vi "Heat2D_Cal Tridiagonal.vi"(9 "Boundary Condition":cluster{"type":T4, "Value":dbl[][]}[](array[cluster]) {"type" items=["Dirichlet", "Neumann"]}, 10 "Coefficients":T2, 11 "Domain":T3={"t"={"initial t"=0.0, "final t"=1.0, "# of t-points"=11}, "x"={"start x"=0.0, "end x"=1.0, "# of x-points"=11}, "y"={"start y"=0.0, "end y"=1.0, "# of y-points"=11}}) -> (0 "X RHS":dbl[][](array[numeric]), 2 "Coefficients Dup":T2, 3 "TriDia Cluster":T1)   [LabVIEW 2017, in "NI_PDE.lvlib"]
uses:
  <vilib>/gmath/NI_PDE.lvlib
  <vilib>/gmath/pde.llb/Common/PDE_BC Type.ctl
  <vilib>/Analysis/NI_AALPro.lvlib
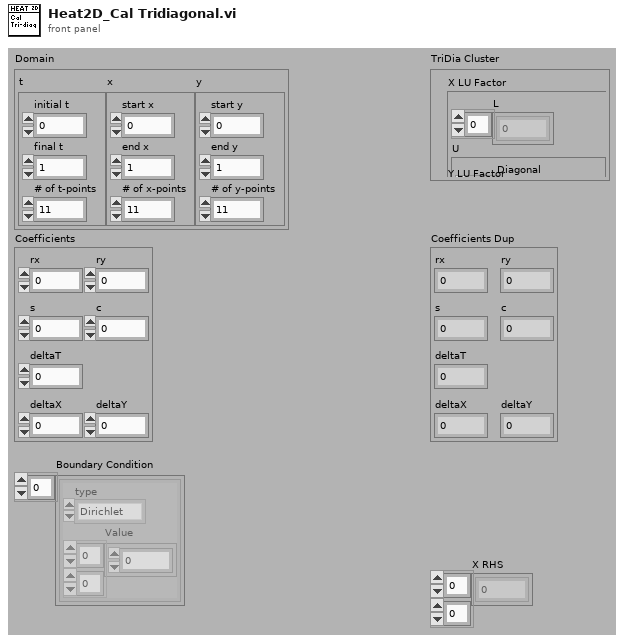
[diagram p1: front panel]
types:
  T1 = cluster{"X LU Factor":cluster{"L":dbl[], "U":cluster{"Diagonal":dbl[], "Super Diagonal":dbl[], "2nd Super Diagonal":dbl[]}, "Pivot":i32[]}, "Y LU Factor":cluster{"L":dbl[], "U":cluster{"Diagonal":dbl[], "Super Diagonal":dbl[], "2nd Super Diagonal":dbl[]}, "Pivot":i32[]}, "X Tridiagonal":cluster{"SubDiagonal":dbl[], "MainDiagonal":dbl[], "SuperDiagonal":dbl[]}, "Y Tridiagonal":cluster{"SubDiagonal":dbl[], "MainDiagonal":dbl[], "SuperDiagonal":dbl[]}}
  T2 = cluster{"rx":dbl, "ry":dbl, "s":dbl, "c":dbl, "deltaT":dbl, "deltaX":dbl, "deltaY":dbl}
  T3 = cluster{"t":cluster{"initial t":dbl, "final t":dbl, "# of t-points":i32}, "x":cluster{"start x":dbl, "end x":dbl, "# of x-points":i32}, "y":cluster{"start y":dbl, "end y":dbl, "# of y-points":i32}}
  T4 = typedef "NI_PDE.lvlib/PDE_BC Type.ctl" = i32
  T5 = cluster{"SubDiagonal":dbl[], "MainDiagonal":dbl[], "SuperDiagonal":dbl[]}
  T6 = cluster{"Diagonal":dbl[], "Super Diagonal":dbl[], "2nd Super Diagonal":dbl[]}
  T7 = cluster{"L":dbl[], "U":cluster{"Diagonal":dbl[], "Super Diagonal":dbl[], "2nd Super Diagonal":dbl[]}, "Pivot":i32[]}
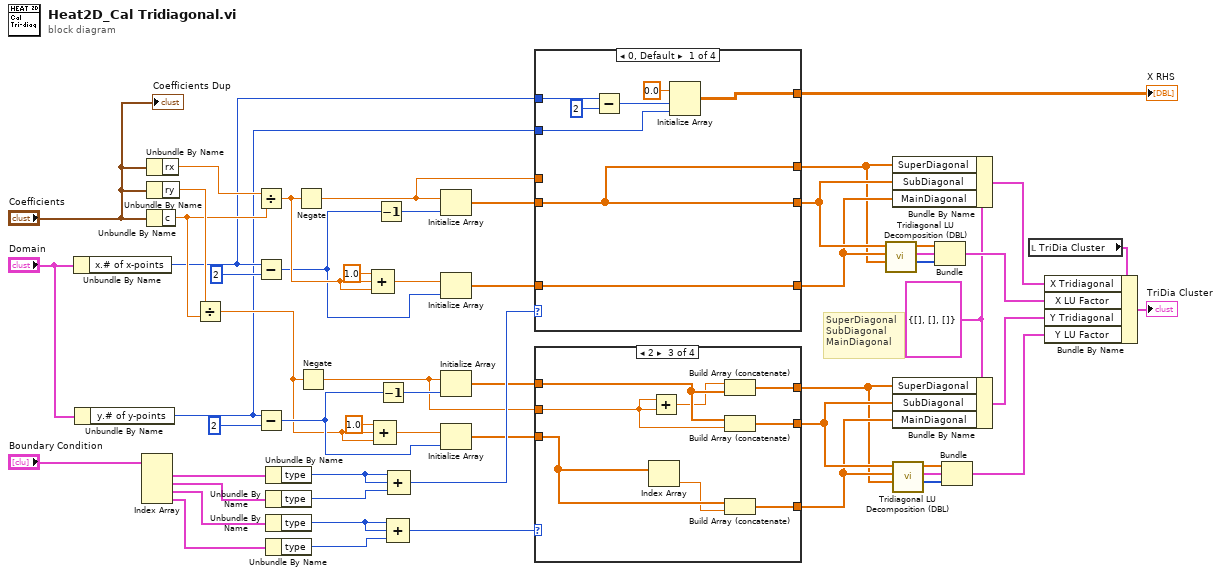
[diagram p0: block diagram]
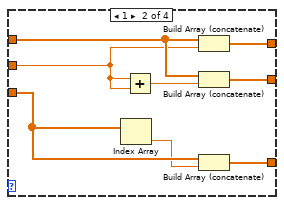
[diagram p3: hidden frame]
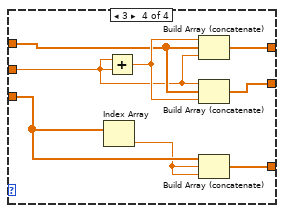
[diagram p4: hidden frame]
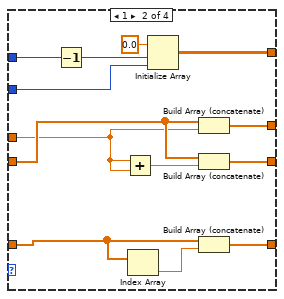
[diagram p5: hidden frame]
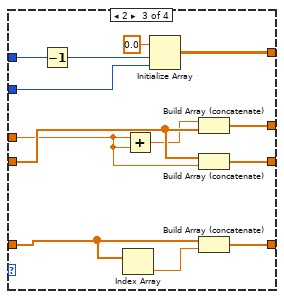
[diagram p6: hidden frame]
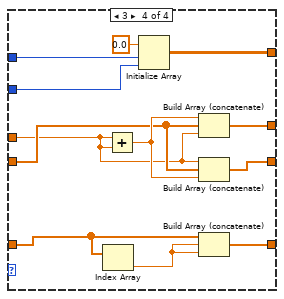
[diagram p7: hidden frame]
diagram:
  w2 = T5 {"SubDiagonal"=[], "MainDiagonal"=[], "SuperDiagonal"=[]} ("Tridiagonals")
  # "SuperDiagonal\nSubDiagonal\nMainDiagonal"
  n1 = Unbundle By Name("Domain") -> ("x.# of x-points"=w5:i32)
  n2 = Unbundle By Name("Domain") -> ("y.# of y-points"=w1:i32)
  n3 = Index Array(array="Boundary Condition") -> (element #1=w49:cluster{"type":T4, "Value":dbl[][]}, element #2=w48:cluster{"type":T4, "Value":dbl[][]}, element #3=w47:cluster{"type":T4, "Value":dbl[][]}, element #4=w46:cluster{"type":T4, "Value":dbl[][]})  [unwired: 4 in]
  n4 = Unbundle By Name("Coefficients") -> ("rx"=w26:dbl)
  n5 = Unbundle By Name("Coefficients") -> ("ry"=w29:dbl)
  n6 = Unbundle By Name("Coefficients") -> ("c"=w27:dbl)
  n7 = Divide(x=w29, y=w27) -> (x/y=w38:dbl)
  n8 = Divide(x=w26, y=w27) -> (x/y=w54:dbl)
  n9 = Subtract(x=w5, y=2) -> (x-y=w51:i32)
  n10 = Subtract(x=w1, y=2) -> (x-y=w43:i32)
  n11 = Unbundle By Name(w49) -> ("type"=w45:T4)
  n12 = Unbundle By Name(w48) -> ("type"=w44:T4)
  n13 = Unbundle By Name(w47) -> ("type"=w34:T4)
  n14 = Unbundle By Name(w46) -> ("type"=w33:T4)
  n15 = Negate(x=w54) -> (-x=w25:dbl)
  n16 = Negate(x=w38) -> (-x=w24:dbl)
  n17 = Compound Arithmetic op=ADD(1.0 ("value"), w54, w54) -> (w52:dbl)
  n18 = Compound Arithmetic op=ADD(1.0 ("value"), w38, w38) -> (w42:dbl)
  n19 = Decrement(x=w51) -> (x-1=w55:i32)
  n20 = Decrement(x=w43) -> (x-1=w40:i32)
  n21 = Compound Arithmetic op=ADD(w34, w34, w33) -> (w30:T4)
  n22 = Compound Arithmetic op=ADD(w45, w45, w44) -> (w37:T4)
  n23 = Initialize Array(w25, w55) -> (w36:dbl[])
  n24 = Initialize Array(w52, w51) -> (w35:dbl[])
  n25 = Initialize Array(w24, w40) -> (w32:dbl[])
  n26 = Initialize Array(w42, w43) -> (w31:dbl[])
  n27 = case shown="0, Default" w37 {
    tunnel: w36 -> [w63 w75 w87 w98]
    tunnel: w35 -> [w64 w71 w84 w96]
    tunnel: [w63 w76 w89 w101] -> w23
    tunnel: [w64 w73 w88 w100] -> w22
    tunnel: [w63 w77 w90 w102] -> w21
    tunnel: w25 -> [_ w72 w85 w97]
    tunnel: w5 -> [w62 w67 w81 w93]
    tunnel: w1 -> [w59 w66 w79 w92]
    tunnel: [w57 w65 w78 w91] -> w3
    frame 0, Default {
      n28 = Subtract(x=w62, y=2) -> (x-y=w60:i32)
      n29 = Initialize Array(0.0 ("element"), w60, w59) -> (w57:dbl[][])
    }
    frame 1 {
      n30 = Decrement(x=w67) -> (x-1=w68:i32)
      n31 = Add(x=w72, y=w72) -> (x+y=w74:dbl)
      n32 = Index Array(array=w71) -> (element=w70:dbl)  [unwired: 1 in]
      n33 = Initialize Array(0.0 ("element"), w68, w66) -> (w65:dbl[][])
      n34 = Build Array (concatenate)(w75, w72) -> (w77:dbl[])
      n35 = Build Array (concatenate)(w75, w74) -> (w76:dbl[])
      n36 = Build Array (concatenate)(w71, w70) -> (w73:dbl[])
    }
    frame 2 {
      n37 = Decrement(x=w81) -> (x-1=w80:i32)
      n38 = Index Array(array=w84) -> (element=w83:dbl)  [unwired: 1 in]
      n39 = Add(x=w85, y=w85) -> (x+y=w86:dbl)
      n40 = Initialize Array(0.0 ("element"), w80, w79) -> (w78:dbl[][])
      n41 = Build Array (concatenate)(w86, w87) -> (w90:dbl[])
      n42 = Build Array (concatenate)(w87, w85) -> (w89:dbl[])
      n43 = Build Array (concatenate)(w84, w83) -> (w88:dbl[])
    }
    frame 3 {
      n44 = Index Array(array=w96) -> (element=w95:dbl)  [unwired: 1 in]
      n45 = Add(x=w97, y=w97) -> (x+y=w99:dbl)
      n46 = Initialize Array(0.0 ("element"), w93, w92) -> (w91:dbl[][])
      n47 = Build Array (concatenate)(w99, w98, w97) -> (w102:dbl[])
      n48 = Build Array (concatenate)(w97, w98, w99) -> (w101:dbl[])
      n49 = Build Array (concatenate)(w96, w95, w95) -> (w100:dbl[])
    }
  }
  "X RHS" <- w3
  n50 = case shown="2" w30 {
    tunnel: w32 -> [w103 w110 w117 w124]
    tunnel: w31 -> [w104 w106 w114 w122]
    tunnel: [w103 w111 w119 w127] -> w14
    tunnel: [w104 w108 w118 w126] -> w13
    tunnel: [w103 w112 w120 w128] -> w12
    tunnel: w24 -> [_ w107 w115 w123]
    frame 0, Default {
    }
    frame 1 {
      n51 = Index Array(array=w106) -> (element=w105:dbl)  [unwired: 1 in]
      n52 = Add(x=w107, y=w107) -> (x+y=w109:dbl)
      n53 = Build Array (concatenate)(w110, w107) -> (w112:dbl[])
      n54 = Build Array (concatenate)(w110, w109) -> (w111:dbl[])
      n55 = Build Array (concatenate)(w106, w105) -> (w108:dbl[])
    }
    frame 2 {
      n56 = Index Array(array=w114) -> (element=w113:dbl)  [unwired: 1 in]
      n57 = Add(x=w115, y=w115) -> (x+y=w116:dbl)
      n58 = Build Array (concatenate)(w116, w117) -> (w120:dbl[])
      n59 = Build Array (concatenate)(w117, w115) -> (w119:dbl[])
      n60 = Build Array (concatenate)(w114, w113) -> (w118:dbl[])
    }
    frame 3 {
      n61 = Index Array(array=w122) -> (element=w121:dbl)  [unwired: 1 in]
      n62 = Add(x=w123, y=w123) -> (x+y=w125:dbl)
      n63 = Build Array (concatenate)(w125, w124, w123) -> (w128:dbl[])
      n64 = Build Array (concatenate)(w123, w124, w125) -> (w127:dbl[])
      n65 = Build Array (concatenate)(w122, w121, w121) -> (w126:dbl[])
    }
  }
  n66 = call <vilib>:"Tridiagonal LU Decomposition (DBL).vi"("Super Diagonal"=w21, "Diagonal"=w22, "Sub Diagonal"=w23) -> ("Pivot"=w18:i32[], "U"=w19:T6, "L"=w20:dbl[])  [unwired: 6 out]
  n67 = Bundle By Name(cluster=w2, "SuperDiagonal"=w21, "SubDiagonal"=w23, "MainDiagonal"=w22) -> (w9:T5)
  n68 = Bundle By Name(cluster=w2, "SuperDiagonal"=w12, "SubDiagonal"=w14, "MainDiagonal"=w13) -> (w7:T5)
  n69 = call <vilib>:"Tridiagonal LU Decomposition (DBL).vi"("Super Diagonal"=w12, "Diagonal"=w13, "Sub Diagonal"=w14) -> ("Pivot"=w17:i32[], "U"=w16:T6, "L"=w15:dbl[])  [unwired: 6 out]
  n70 = Bundle("L"=w20, "U"=w19, "Pivot"=w18) -> (w8:T7)  [unwired: 1 out]
  n71 = Bundle("L"=w15, "U"=w16, "Pivot"=w17) -> (w6:T7)  [unwired: 1 out]
  n72 = local read "TriDia Cluster"() -> (w10:T1)
  n73 = Bundle By Name(cluster=w10, "X Tridiagonal"=w9, "X LU Factor"=w8, "Y Tridiagonal"=w7, "Y LU Factor"=w6) -> (→"TriDia Cluster":T1)
  "Coefficients Dup" <- "Coefficients"
